vi "Add Channels.vi"(8 "error in (no error)":errorcluster, 10 "Channels Setup":T3(array[cluster]), 11 "Section Ptr In":T4 format="%.0x") -> (0 "error out":errorcluster, 3 "Section Ptr Out":T4 format="%.0x")   [LabVIEW 2020, in "Vires VTD System Explorer.lvlib"]
uses:
  Vires VTD System Explorer.lvlib
  <vilib>/NI VeriStand/Custom Device API/Custom Device Item Ref.ctl
  <vilib>/NI VeriStand/Custom Device API/Custom Device Channel.ctl
  <vilib>/NI VeriStand/Custom Device API/Custom Device Channel Type.ctl
  Shared/Constants.vi
  <vilib>/NI VeriStand/Custom Device API/Custom Device API.lvlib
  Shared/Vires VTD Shared.lvlib
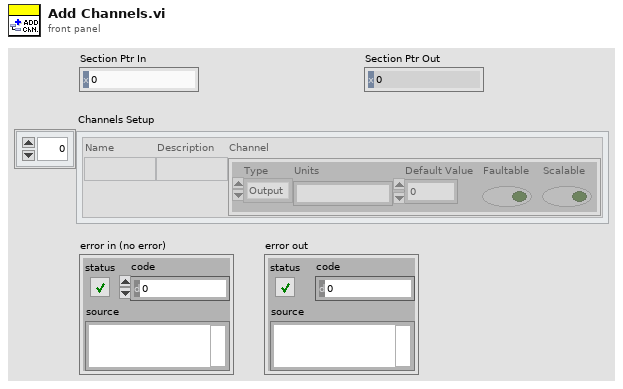
[diagram p1: front panel]
types:
  T1 = typedef "Custom Device API.lvlib/Custom Device Channel.ctl" = cluster{"Type":T2, "Units":string, "Default Value":dbl, "Faultable":bool, "Scalable":bool}
  T2 = typedef "Custom Device API.lvlib/Custom Device Channel Type.ctl" = enum16{"Input", "Output"}
  T3 = cluster{"Name":string, "Description":string, "Channel":T1}[]
  T4 = typedef "Custom Device API.lvlib/Custom Device Item Ref.ctl" = u64
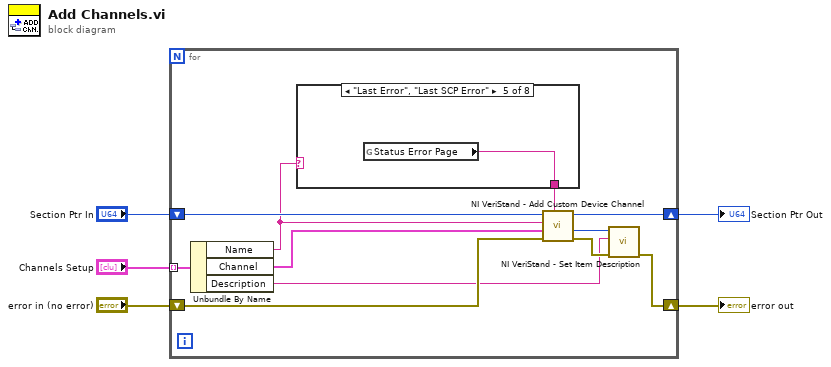
[diagram p0: block diagram]
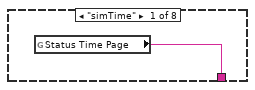
[diagram p2: hidden frame]
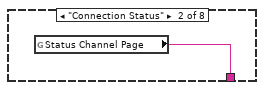
[diagram p3: hidden frame]
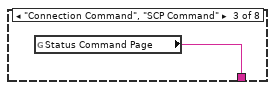
[diagram p4: hidden frame]
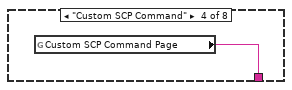
[diagram p5: hidden frame]
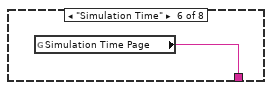
[diagram p6: hidden frame]
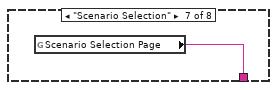
[diagram p7: hidden frame]
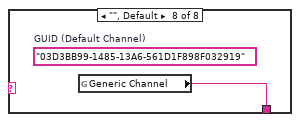
[diagram p8: hidden frame]
diagram:
  n1 = for {
    shift-right: [w12] -> w4
    shift-left: "error in (no error)" -> [w15]
    tunnel: "Channels Setup" -> [w10] mode=indexing
    shift-right: [w11] -> w1
    shift-left: "Section Ptr In" -> [w16]
    n2 = Unbundle By Name(w10) -> ("Name"=w7:string, "Channel"=w8:T1, "Description"=w9:string)
    n3 = case shown="\"Last Error\", \"Last SCP Error\"" w7 {
      tunnel: [w17 w18 w19 w20 w21 w22 w23 w24] -> w6
      frame "simTime" {
        n4 = global read "Constants.vi" "Status Time Page"() -> (w17:string)
      }
      frame "Connection Status" {
        n5 = global read "Constants.vi" "Status Channel Page"() -> (w18:string)
      }
      frame "Connection Command", "SCP Command" {
        n6 = global read "Constants.vi" "Status Command Page"() -> (w19:string)
      }
      frame "Custom SCP Command" {
        n7 = global read "Constants.vi" "Custom SCP Command Page"() -> (w20:string)
      }
      frame "Last Error", "Last SCP Error" {
        n8 = global read "Constants.vi" "Status Error Page"() -> (w21:string)
      }
      frame "Simulation Time" {
        n9 = global read "Constants.vi" "Simulation Time Page"() -> (w22:string)
      }
      frame "Scenario Selection" {
        n10 = global read "Constants.vi" "Scenario Selection Page"() -> (w23:string)
      }
      frame "", Default {
        (unwired) "03D3BB99-1485-13A6-561D1F898F032919"  # GUID (Default Channel)
        n11 = global read "Constants.vi" "Generic Channel"() -> (w24:string)
      }
    }
    n12 = call <vilib>:"NI VeriStand - Add Custom Device Channel.vi"("GUID (Default Channel)"=w6, "error in (no error)"=w15, "Channel"=w8, "Channel Name"=w7, "Parent Ref in"=w16) -> ("error out"=w14:errorcluster, "Channel Ref"=w13:T4, "Parent Ref out"=w11:T4)  [unwired: 3 in, 1 out]
    n13 = call <vilib>:"NI VeriStand - Set Item Description.vi"("error in (no error)"=w14, "Description"=w9, "Item Ref in"=w13) -> ("error out"=w12:errorcluster)  [unwired: 6 in, 2 out]
  }
  "error out" <- w4
  "Section Ptr Out" <- w1
